vi "SetAttributeViBoolean_SA-Limit_Mask.vi"(7 "AttributeValue (Off)":bool, 8 "error in (no error)":errorcluster {"code" format="%.0x"}, 9 "AttributeID":u32(ring)=1150619 items=["SA_LIMIT_DISPLAY_ENABLED"=1150619, "SA_LIMIT_ENABLED"=1150621, "SA_LIMIT_LINE_ENABLED"=1150745, "SA_LIMIT_MARGIN_ENABLED"=1150625, "SA_LIMIT_REALTIVE_TO_CENTER_FREQUENCY_ENABLED"=1150627, "SA_LIMIT_RELATIVE_TO_AMPLITUDE_ENABLED"=1150628, "SA_SEMASK_AVERAGE_ENABLED"=1150360, "SA_SEMASK_DISPLAY_LIMIT_LINE_ENABLED"=1150397, "SA_SEMASK_DISPLAY_WINDOWX_AUTO_SCALE_ENABLED"=1150817, "SA_SEMASK_DISPLAY_WINDOWY_AUTO_SCALE_ENABLED"=1150384, "SA_SEMASK_MARKER_COUPLE_ENABLED"=1150402, "SA_SEMASK_MARKER_ENABLED"=1150404, "SA_SEMASK_OFFSET_DETECTOR_TYPE_AUTO_ENABLED"=1150409, "SA_SEMASK_OFFSETFILTER_ENABLED"=1150382, "SA_SEMASK_REFERENCECHANNEL_DETECTOR_TYPE_AUTO_ENABLED"=1150366, "SA_SEMASK_REFERENCECHANNEL_TOTAL_POWER_AUTO_ENABLED"=1150364, "SA_SEMASK_SWEEPCOUPLING_BANDWIDTH_RATIO_AUTO_ENABLED"=1150377, "SA_SEMASK_SWEEPCOUPLING_RESOLUTION_BANDWIDTH_AUTO_ENABLED"=1150373, "SA_SEMASK_SWEEPCOUPLING_SWEEP_TIME_AUTO_ENABLED"=1150376, "SA_SEMASK_SWEEPCOUPLING_SWEEP_TYPE_AUTO_ENABLED"=1150819, "SA_SEMASK_SWEEPCOUPLING_VIDEO_BANDWIDTH_AUTO_ENABLED"=1150379], 10 "RepCapIdentifier":string, 11 "instrument handle":refnum<k15>) -> (0 "error out":errorcluster {"code" format="%.0x"}, 3 "instrument handle out":refnum<k15>)   [LabVIEW 2009, in "Keysight XSAn.lvlib"]
doc: "Sets a Boolean attribute from the instrument driver.\nThe following Attributes are supported:\n\nSA_LIMIT_DISPLAY_ENABLED\nSA_LIMIT_ENABLED\nSA_LIMIT_LINE_ENABLED\nSA_LIMIT_MARGIN_ENABLED\nSA_LIMIT_REALTIVE_TO_CENTER_FREQUENCY_ENABLED\nSA_LIMIT_RELATIVE_TO_AMPLITUDE_ENABLED\nSA_SEMASK_AVERAGE_ENABLED\nSA_SEMASK_DISPLAY_LIMIT_LINE_ENABLED\nSA_SEMASK_DISPLAY_WINDOWX_AUTO_SCALE_ENABLED \nSA_SEMASK_DISPLAY_WINDOWY_AUTO_SCALE_ENABLED\nSA_SEMASK_MARKER_COUPLE_ENABLED\nSA_SEMASK_MARKER_ENABLED\nSA_SEMASK_OFFSET_DETECTOR_TYPE_AUTO_ENABLED\nSA_SEMASK_OFFSETFILTER_ENABLED\nSA_SEMASK_REFERENCECHANNEL_DETECTOR_TYPE_AUTO_ENABLED\nSA_SEMASK_REFERENCECHANNEL_TOTAL_POWER_AUTO_ENABLED\nSA_SEMASK_SWEEPCOUPLING_BANDWIDTH_RATIO_AUTO_ENABLED\nSA_SEMASK_SWEEPCOUPLING_RESOLUTION_BANDWIDTH_AUTO_ENABLED\nSA_SEMASK_SWEEPCOUPLING_SWEEP_TIME_AUTO_ENABLED\nSA_SEMASK_SWEEPCOUPLING_SWEEP_TYPE_AUTO_ENABLED \nSA_SEMASK_SWEEPCOUPLING_VIDEO_BANDWIDTH_AUTO_ENABLED"
uses:
  <instrlib>/Keysight XSAn/Keysight XSAn.lvlib
  AgXSAn.dll
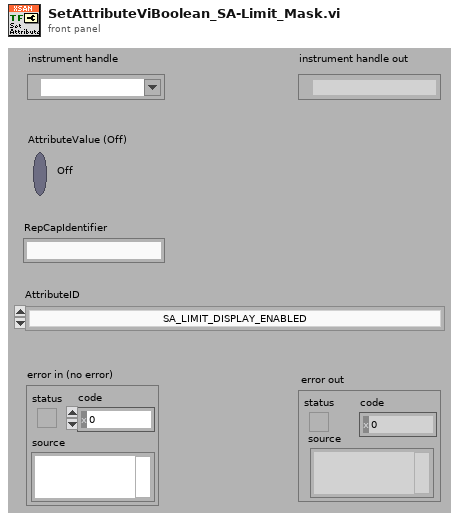
[diagram p1: front panel]
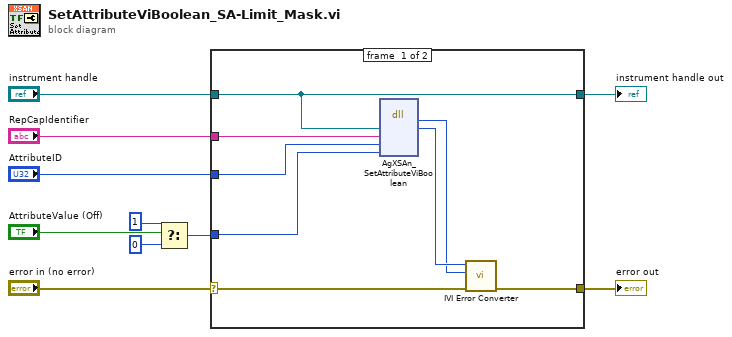
[diagram p0: block diagram]
diagram:
  n1 = Select(t=u16 1, s="AttributeValue (Off)", f=u16 0) -> (s? t:f=w2:u16)
  n2 = case shown="No Error" "error in (no error)" {
    selector: "error in (no error)" -> [w16 w20]
    tunnel: [w15 w20] -> w10
    tunnel: "instrument handle" -> [w11 w19]
    tunnel: "RepCapIdentifier" -> [w14 _]
    tunnel: "AttributeID" -> [w13 _]
    tunnel: w2 -> [w12 _]
    tunnel: [w11 w19] -> w1
    frame #0 {
      n3 = dll-call lib="AgXSAn**.dll" fn="AgXSAn_SetAttributeViBoolean"("Vi"=w11, "RepCapIdentifier"=w14, "AttributeID"=w13, "AttributeValue"=w12) -> ("return type"=w17:i32, "Vi"=w18:u32)  [unwired: 6 in, 2 out]
      n4 = call <instrlib>:"IVI Error Converter.vi"("error in (no error)"=w16, "IVI error code (0)"=w17, "instrument handle"=w18) -> ("error out"=w15:errorcluster)  [unwired: 7 in, 1 out]
    }
    frame #1 {
    }
  }
  "error out" <- w10
  "instrument handle out" <- w1
